vi "Receive Value Change Event.vi"(8 "error in (no error)":errorcluster, 10 "ValueChangeMsg":refnum<class "ValueChangeMsg.lvclass">, 11 "For Loop Dialog In":refnum<class "Test Step Dialog.lvclass">) -> (0 "error out":errorcluster, 3 "For Loop Dialog Out":refnum<class "Test Step Dialog.lvclass">)   [LabVIEW 2017, in "Test Step Dialog.lvclass"]
doc: "<License>\nCopyright © 2017 Composed Systems, LLC | All rights reserved\nwww.composed.io\n\nAuthor: Ethan Stern <ethan.stern@composed.io>\n\nThis software is provided \"AS IS\" WITHOUT WARRANTIES, either express or implied, AND IS FOR EDUCATIONAL PURPOSES ONLY.\n</License>"
uses:
  Test Step Dialog.lvclass
  C:/Program Files/National Instruments/LabVIEW 2017/vi.lib/ActorFramework/Actor/Actor.lvclass
  C:/Program Files/National Instruments/LabVIEW 2017/vi.lib/gpm_packages/@cs/popup-viewmanager/Source/Popup ViewManager/Popup ViewManager.lvclass
  D:/Test-executive-builder/Source/Test Executive Builder Dialogs/ITest Executive Builder Dialog/ITest Executive Builder Dialog.lvclass
  <vilib>/gpm_packages/@cs/mva-viewable/Source/ActorEvents/IEventAggregator Messages/ValueChangeMsg/ValueChangeMsg.lvclass
  <vilib>/gpm_packages/@cs/mva-viewable/Source/ActorEvents/IEventAggregator Messages/ValueChangeMsg/ValueChangeMsg.lvclass/ValueChangeMsg.ctl
  Data Type Handler/Test Executive Builder Data Type Handler.lvclass
  <vilib>/ActorFramework/Actor/Actor.lvclass/Actor.ctl
  <vilib>/ActorFramework/Message Enqueuer/Message Enqueuer.lvclass/Message Enqueuer.ctl
  Test Step Dialog.lvclass/Test Step Dialog.ctl
  <vilib>/gpm_packages/@cs/mva-viewable/Source/IViewable/IViewable Messages/Insert Front Panel Msg/Insert Front Panel Msg.lvclass/Insert Front Panel Msg.ctl
  IAttribute Data Type View Messages/Set Value Msg/Set Value Msg.lvclass/Set Value Msg.ctl
  ITest Executive Builder Dialog/ITest Executive Builder Dialog.lvclass/ITest Executive Builder Dialog.ctl
  698eee39-0e44-4932-ada2-d875f71f8c5a.vi
  7755fdff-7f77-4a95-a937-83a1493eaaf5.vi
  482c0f58-527f-4f41-8bf0-1e92f0d36b0a.vi
  <vilib>/ActorFramework/Message Enqueuer/Init from Existing Queue.vi
  <vilib>/ActorFramework/Message Enqueuer/Enqueue.vi
  ITest Executive Builder Dialog/Read Data Type Handler Type.vi
  <vilib>/Utility/error.llb/Clear Errors.vi
  <vilib>/ActorFramework/Stop Msg/Stop Msg.lvclass
  C:/Program Files/National Instruments/LabVIEW 2017/vi.lib/ActorFramework/Message/Message.lvclass
  <vilib>/gpm_packages/@cs/mva-viewable/Source/IViewable/IViewable Messages/Insert Front Panel Msg/Insert Front Panel Msg.lvclass
  IAttribute Data Type View Messages/Set Value Msg/Set Value Msg.lvclass
  <vilib>/ActorFramework/Message Priority Queue/Priority Enqueue.vi
  <vilib>/ActorFramework/Message Enqueuer/Message Enqueuer.lvclass
  <vilib>/gpm_packages/@cs/test-executive/Source/Test Executive/ITestExecutive/ITest Executive.lvclass
  ITest Executive Builder Dialog/ITest Executive Builder Dialog.lvclass
  <vilib>/ActorFramework/Actor/Actor.lvclass
  <vilib>/gpm_packages/@cs/popup-viewmanager/Source/Popup ViewManager/Popup ViewManager.lvclass
  <vilib>/gpm_packages/@cs/test-executive/Source/Test Executive/TestExecutive Ref/TestExecutive Ref.lvclass
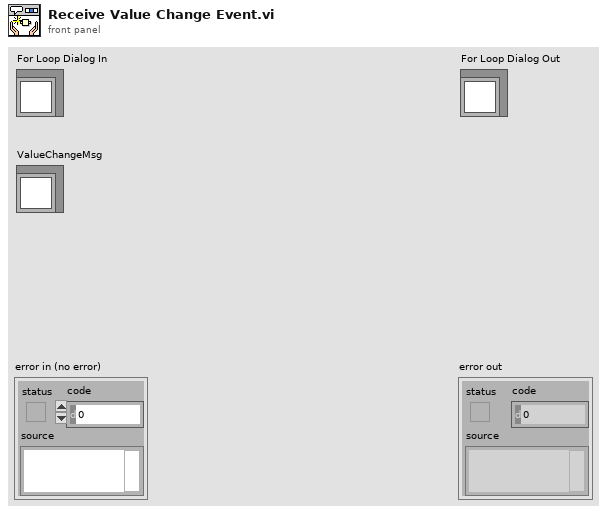
[diagram p1: front panel]
types:
  T1 = typedef "IViewable.lvlib/ProtectedSubpanel.lvclass/Protected Subpanel Reference.ctl" = refnum<data-value>
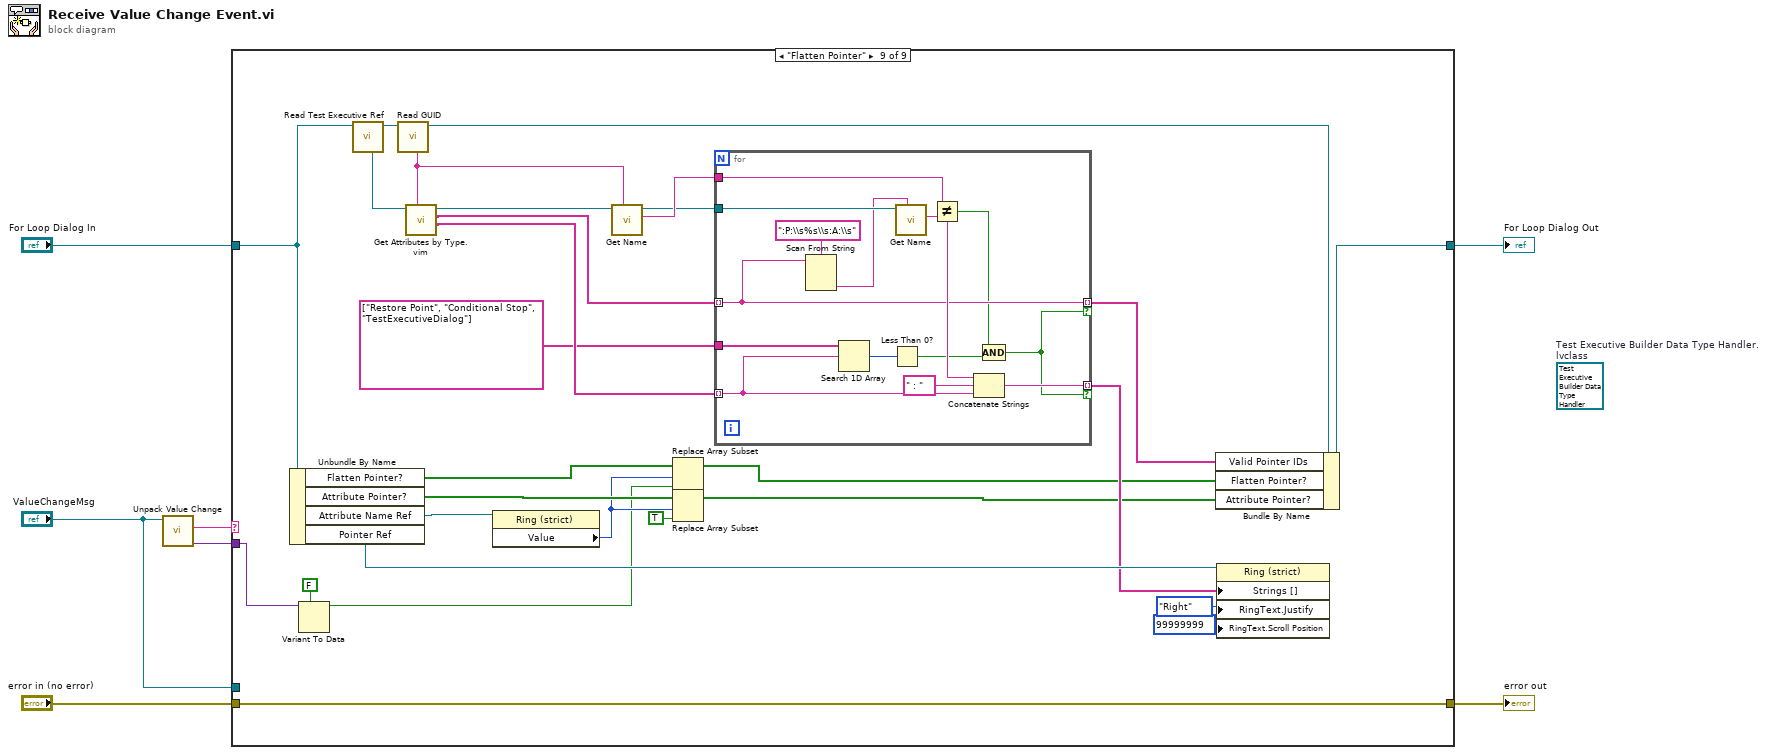
[diagram p0: block diagram]
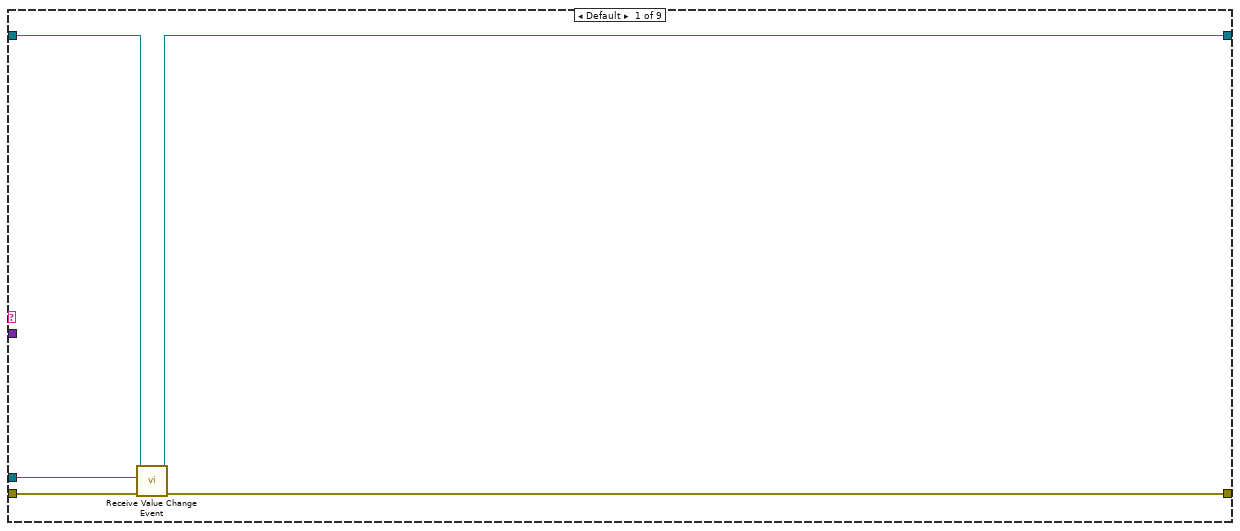
[diagram p2: hidden frame]
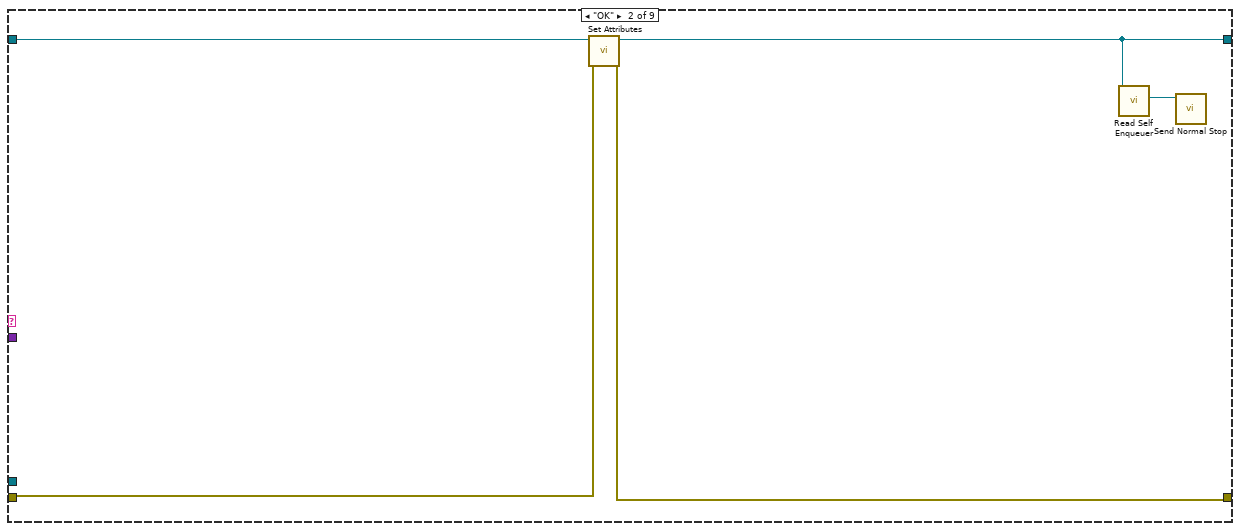
[diagram p3: hidden frame]
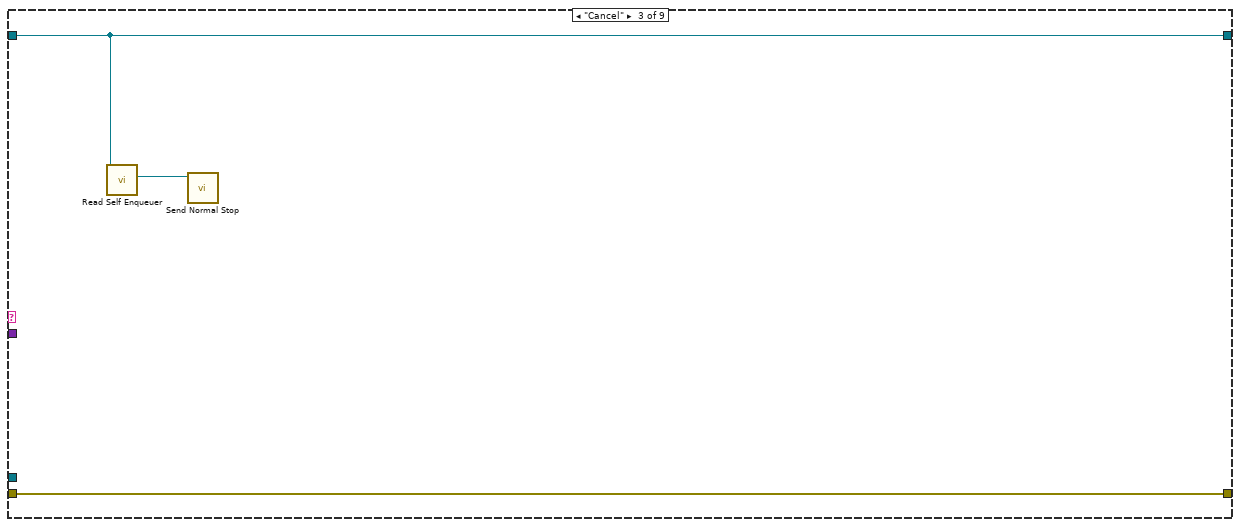
[diagram p4: hidden frame]
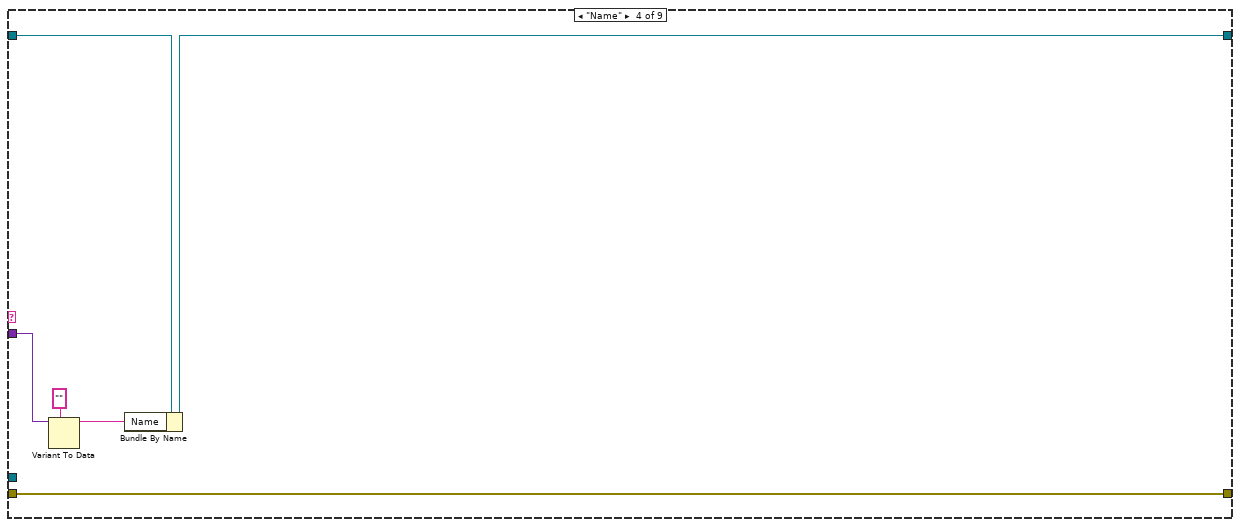
[diagram p5: hidden frame]
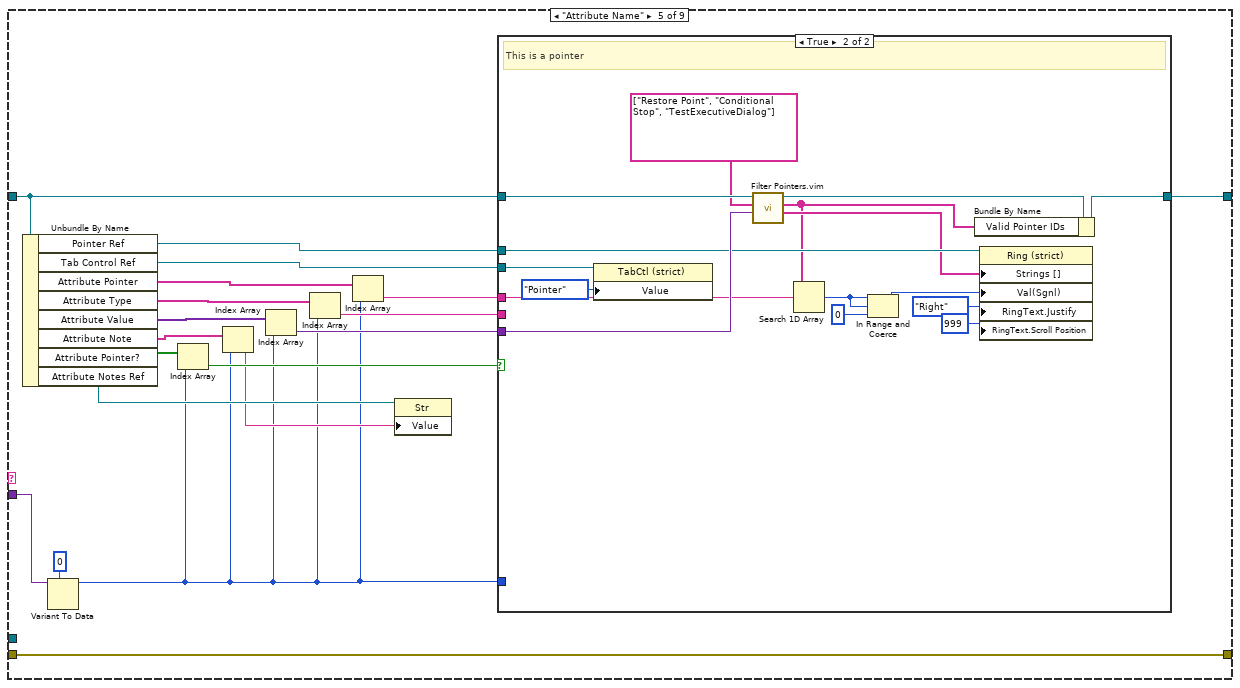
[diagram p6: hidden frame]
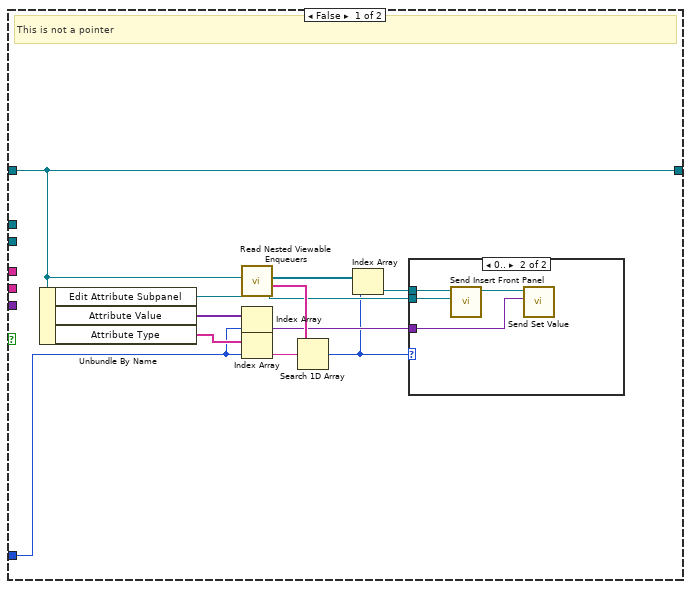
[diagram p7: hidden frame]
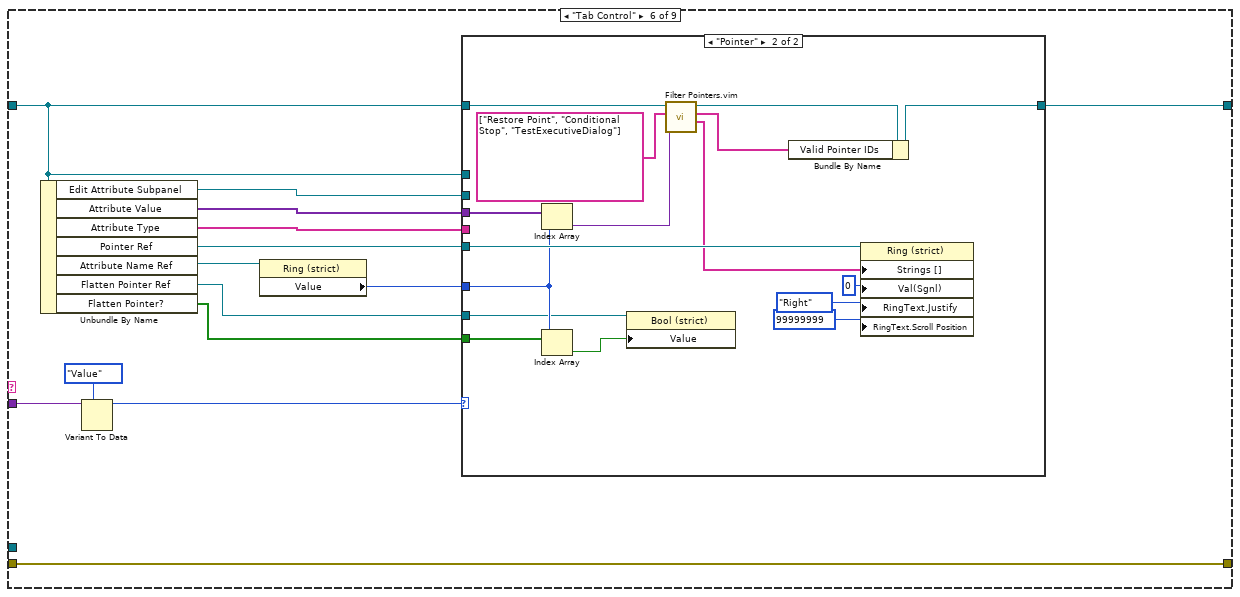
[diagram p9: hidden frame]
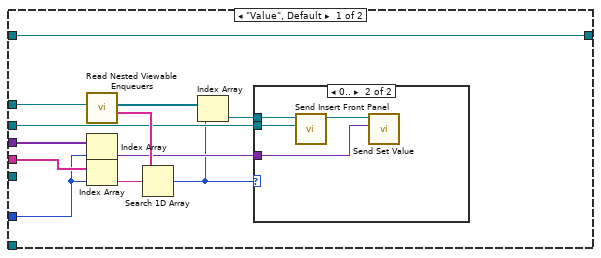
[diagram p10: hidden frame]
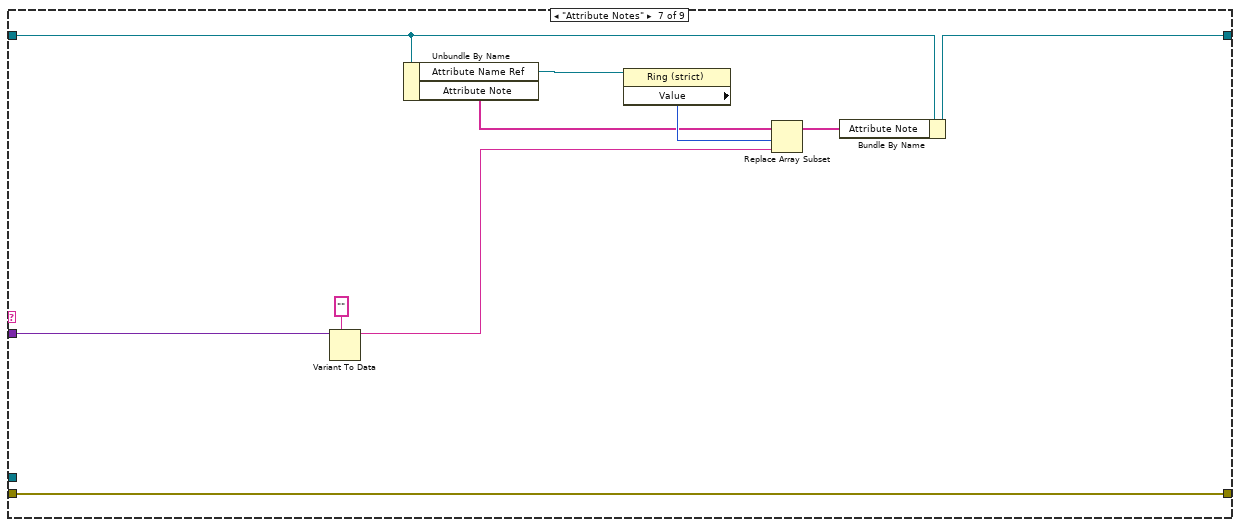
[diagram p12: hidden frame]
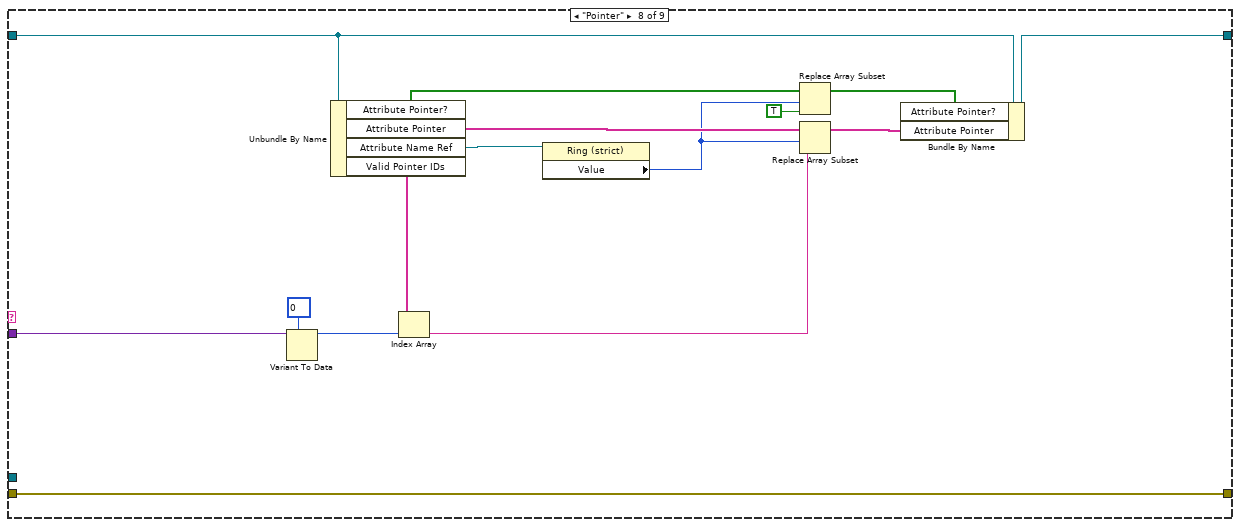
[diagram p13: hidden frame]
diagram:
  (unwired) refnum<class "Test Executive Builder Data Type Handler.lvclass"> refnum  # Test Executive Builder Data Type Handler.lvclass
  n1 = call <vilib>:"Unpack Value Change.vi"("ValueChangeMsg"="ValueChangeMsg") -> ("New Value"=w1:variant, "Control Label"=w2:string)  [unwired: 6 in, 3 out]
  n2 = case shown="\"Flatten Pointer\"" w2 {
    tunnel: [w12 w13 w20 w26 w45 w90 w132 w147 w175] -> w7
    tunnel: [w11 w15 w19 w21 w44 w86 w124 w134 w158] -> w6
    tunnel: "error in (no error)" -> [w10 w14 w20 w26 w45 w90 w132 w147 w175]
    tunnel: "For Loop Dialog In" -> [w9 w16 w19 w22 w43 w79 w125 w135 w173]
    tunnel: "ValueChangeMsg" -> [w8 _ _ _ _ _ _ _ _]
    tunnel: w1 -> [_ _ _ w25 w42 w89 w123 w133 w151]
    frame Default {
      n3 = call-parent "Receive Value Change Event.vi"("error in (no error)"=w10, "ValueChangeMsg"=w8, "IViewable In"=w9) -> ("error out"=w12:errorcluster, "IViewable Out"=w11:refnum<class "Test Step Dialog.lvclass">)  [unwired: 7 in]
    }
    frame "OK" {
      n4 = call-dynamic "Set Attributes.vi"("error in (no error)"=w14, "Test Step Dialog in"=w16) -> ("error out"=w13:errorcluster, "Test Step Dialog out"=w15:refnum<class "Test Step Dialog.lvclass">)  [unwired: 8 in]
      n5 = call <vilib>:"Read Self Enqueuer.vi"("Actor"=w15) -> ("Self Enqueuer"=w17:refnum<class "Message Enqueuer.lvclass">)  [unwired: 10 in]
      n6 = call <vilib>:"Send Normal Stop.vi"("Message Enqueuer"=w17) -> ()  [unwired: 10 in, 1 out]
    }
    frame "Cancel" {
      n7 = call <vilib>:"Read Self Enqueuer.vi"("Actor"=w19) -> ("Self Enqueuer"=w18:refnum<class "Message Enqueuer.lvclass">)  [unwired: 10 in]
      n8 = call <vilib>:"Send Normal Stop.vi"("Message Enqueuer"=w18) -> ()  [unwired: 10 in, 1 out]
    }
    frame "Name" {
      n9 = Variant To Data(type="" ("Iterations"), Variant=w25) -> (data=w23:string)  [unwired: 1 in, 1 out]
      n10 = Bundle By Name(cluster=w22, "Name"=w23) -> (w21:refnum<class "Test Step Dialog.lvclass">)
    }
    frame "Attribute Name" {
      n11 = Unbundle By Name(w43) -> ("Pointer Ref"=w30:refnum<vi>, "Tab Control Ref"=w31:refnum<vi>, "Attribute Pointer"=w36:string[], "Attribute Type"=w37:string[], "Attribute Value"=w38:variant[], "Attribute Note"=w39:string[], "Attribute Pointer?"=w40:bool[], "Attribute Notes Ref"=w29:refnum<vi>)
      n12 = Variant To Data(type=u16 0, Variant=w42) -> (data=w27:u16)  [unwired: 1 in, 1 out]
      n13 = Index Array(array=w40, index=w27) -> (element=w35:bool)
      n14 = Index Array(array=w39, index=w27) -> (element=w28:string)
      n15 = Index Array(array=w38, index=w27) -> (element=w34:variant)
      n16 = Index Array(array=w37, index=w27) -> (element=w33:string)
      n17 = Index Array(array=w36, index=w27) -> (element=w32:string)
      n18 = property class="Str"(reference=w29, "Value"=w28) -> ()  [unwired: 1 in, 2 out]
      n19 = case shown="True" w35 {
        tunnel: [w46 w67] -> w44
        tunnel: w43 -> [w46 w76]
        tunnel: w34 -> [_ w74]
        tunnel: w33 -> [_ _]
        tunnel: w32 -> [_ w65]
        tunnel: w31 -> [_ w73]
        tunnel: w30 -> [_ w72]
        tunnel: w27 -> [w47 _]
        frame False {
          # "This is not a pointer"
          n20 = Unbundle By Name(w46) -> ("Edit Attribute Subpanel"=w50:T1, "Attribute Value"=w55:variant[], "Attribute Type"=w56:string[])
          n21 = call <vilib>:"Read Nested Viewable Enqueuers.vi"("Popup ViewManager in"=w46) -> ("Viewable Names"=w52:string[], "Nested Enqueuers"=w54:refnum<class "Message Enqueuer.lvclass">[])  [unwired: 9 in]
          n22 = Index Array(array=w55, index=w47) -> (element=w49:variant)
          n23 = Index Array(array=w56, index=w47) -> (element=w51:string)
          n24 = Search 1D Array(1D array=w52, element=w51) -> (index of element=w48:i32)  [unwired: 1 in]
          n25 = Index Array(array=w54, index=w48) -> (element=w53:refnum<class "Message Enqueuer.lvclass">)
          n26 = case shown="0.." w48 {
            tunnel: w53 -> [_ w60]
            tunnel: w50 -> [_ w59]
            tunnel: w49 -> [_ w57]
            frame Default {
            }
            frame 0.. {
              n27 = call <vilib>:"Send Insert Front Panel.vi"("Protected Subpanel"=w59, "Message Enqueuer"=w60) -> ("Message Enqueuer out"=w58:refnum<class "Message Enqueuer.lvclass">)  [unwired: 8 in, 1 out]
              n28 = call "Send Set Value.vi"("Value"=w57, "Message Enqueuer"=w58) -> ()  [unwired: 8 in, 2 out]
            }
          }
        }
        frame True {
          # "This is a pointer"
          n29 = property class="TabCtl (strict)"(reference=w73, "Value"=enum32{"Value", "Pointer"}."Pointer") -> ()  [unwired: 1 in, 2 out]
          n30 = call "Filter Pointers.vim"("Type"=w74, "Exclusion List"=string[] ["Restore Point", "Conditional Stop", "TestExecutiveDialog"], "ITest Executive Builder Dialog in"=w76) -> ("Valid Pointer Names"=w69:string[], "Valid Pointer IDs"=w66:string[], "ITest Executive Builder Dialog out"=w68:refnum<class "Test Step Dialog.lvclass">)  [unwired: 5 in, 1 out]
          n31 = Search 1D Array(1D array=w66, element=w65) -> (index of element=w64:i32)  [unwired: 1 in]
          n32 = In Range and Coerce(upper limit=w64, x=w64, lower limit=0) -> (coerced(x)=w62:i32)  [unwired: 1 out]
          n33 = Bundle By Name(cluster=w68, "Valid Pointer IDs"=w66) -> (w67:refnum<class "Test Step Dialog.lvclass">)
          n34 = property class="Ring (strict)"(reference=w72, "Strings []"=w69, "Val(Sgnl)"=w62, "RingText.Justify"=enum16{"Left", "Center", "Right"}."Right" ("Ring Text.Justification"), "RingText.Scroll Position"=u32 999 ("Ring Text.Scroll Position")) -> ()  [unwired: 1 in, 2 out]
        }
      }
    }
    frame "Tab Control" {
      n35 = Unbundle By Name(w79) -> ("Edit Attribute Subpanel"=w85:T1, "Attribute Value"=w80:variant[], "Attribute Type"=w81:string[], "Pointer Ref"=w82:refnum<vi>, "Attribute Name Ref"=w87:refnum<vi>, "Flatten Pointer Ref"=w78:refnum<vi>, "Flatten Pointer?"=w77:bool[])
      n36 = Variant To Data(type=enum32{"Value", "Pointer"}."Value" ("Tab Control"), Variant=w89) -> (data=w84:enum32{"Value", "Pointer"})  [unwired: 1 in, 1 out]
      n37 = property class="Ring (strict)"(reference=w87) -> ("Value"=w83:u16)  [unwired: 1 in, 2 out]
      n38 = case shown="\"Pointer\"" w84 {
        tunnel: w81 -> [w102 _]
        tunnel: w80 -> [w101 w121]
        tunnel: w85 -> [w96 _]
        tunnel: w79 -> [w94 _]
        tunnel: w83 -> [w93 w109]
        tunnel: [w91 w115] -> w86
        tunnel: w79 -> [w91 w122]
        tunnel: w82 -> [_ w118]
        tunnel: w78 -> [_ w108]
        tunnel: w77 -> [_ w110]
        frame "Value", Default {
          n39 = call <vilib>:"Read Nested Viewable Enqueuers.vi"("Popup ViewManager in"=w94) -> ("Viewable Names"=w98:string[], "Nested Enqueuers"=w100:refnum<class "Message Enqueuer.lvclass">[])  [unwired: 9 in]
          n40 = Index Array(array=w101, index=w93) -> (element=w95:variant)
          n41 = Index Array(array=w102, index=w93) -> (element=w97:string)
          n42 = Search 1D Array(1D array=w98, element=w97) -> (index of element=w92:i32)  [unwired: 1 in]
          n43 = Index Array(array=w100, index=w92) -> (element=w99:refnum<class "Message Enqueuer.lvclass">)
          n44 = case shown="0.." w92 {
            tunnel: w99 -> [_ w106]
            tunnel: w96 -> [_ w105]
            tunnel: w95 -> [_ w103]
            frame Default {
            }
            frame 0.. {
              n45 = call <vilib>:"Send Insert Front Panel.vi"("Protected Subpanel"=w105, "Message Enqueuer"=w106) -> ("Message Enqueuer out"=w104:refnum<class "Message Enqueuer.lvclass">)  [unwired: 8 in, 1 out]
              n46 = call "Send Set Value.vi"("Value"=w103, "Message Enqueuer"=w104) -> ()  [unwired: 8 in, 2 out]
            }
          }
        }
        frame "Pointer" {
          n47 = Index Array(array=w121, index=w109) -> (element=w120:variant)
          n48 = Index Array(array=w110, index=w109) -> (element=w107:bool)
          n49 = property class="Bool (strict)"(reference=w108, "Value"=w107) -> ()  [unwired: 1 in, 2 out]
          n50 = call "Filter Pointers.vim"("Type"=w120, "Exclusion List"=string[] ["Restore Point", "Conditional Stop", "TestExecutiveDialog"], "ITest Executive Builder Dialog in"=w122) -> ("Valid Pointer Names"=w117:string[], "Valid Pointer IDs"=w114:string[], "ITest Executive Builder Dialog out"=w116:refnum<class "Test Step Dialog.lvclass">)  [unwired: 5 in, 1 out]
          n51 = Bundle By Name(cluster=w116, "Valid Pointer IDs"=w114) -> (w115:refnum<class "Test Step Dialog.lvclass">)
          n52 = property class="Ring (strict)"(reference=w118, "Strings []"=w117, "Val(Sgnl)"=u16 0 ("Value (Signaling)"), "RingText.Justify"=enum16{"Left", "Center", "Right"}."Right" ("Ring Text.Justification"), "RingText.Scroll Position"=u32 99999999 ("Ring Text.Scroll Position")) -> ()  [unwired: 1 in, 2 out]
        }
      }
    }
    frame "Attribute Notes" {
      n53 = Variant To Data(type="", Variant=w123) -> (data=w127:string)  [unwired: 1 in, 1 out]
      n54 = Unbundle By Name(w125) -> ("Attribute Name Ref"=w131:refnum<vi>, "Attribute Note"=w129:string[])
      n55 = property class="Ring (strict)"(reference=w131) -> ("Value"=w130:u16)  [unwired: 1 in, 2 out]
      n56 = Replace Array Subset(array=w129, new element=w127, index=w130) -> (w126:string[])
      n57 = Bundle By Name(cluster=w125, "Attribute Note"=w126) -> (w124:refnum<class "Test Step Dialog.lvclass">)
    }
    frame "Pointer" {
      w146 = u16 0 items=[""] ("Pointer")
      n58 = Variant To Data(type=w146, Variant=w133) -> (data=w138:u16)  [unwired: 1 in, 1 out]
      n59 = Unbundle By Name(w135) -> ("Attribute Pointer?"=w143:bool[], "Attribute Pointer"=w144:string[], "Attribute Name Ref"=w145:refnum<vi>, "Valid Pointer IDs"=w137:string[])
      n60 = Index Array(array=w137, index=w138) -> (element=w136:string)
      n61 = property class="Ring (strict)"(reference=w145) -> ("Value"=w142:u16)  [unwired: 1 in, 2 out]
      n62 = Replace Array Subset(array=w143, new element=TRUE ("new element/subarray"), index=w142) -> (w139:bool[])
      n63 = Replace Array Subset(array=w144, new element=w136, index=w142) -> (w140:string[])
      n64 = Bundle By Name(cluster=w135, "Attribute Pointer?"=w139, "Attribute Pointer"=w140) -> (w134:refnum<class "Test Step Dialog.lvclass">)
    }
    frame "Flatten Pointer" {
      n65 = Unbundle By Name(w173) -> ("Flatten Pointer?"=w153:bool[], "Attribute Pointer?"=w156:bool[], "Attribute Name Ref"=w164:refnum<vi>, "Pointer Ref"=w163:refnum<vi>)
      n66 = Variant To Data(type=FALSE, Variant=w151) -> (data=w149:bool)  [unwired: 1 in, 1 out]
      n67 = call "Read Test Executive Ref.vi"("ITest Executive Builder Dialog in"=w173) -> ("ITest Executive Builder Dialog out"=w174:refnum<class "Test Step Dialog.lvclass">, "Test Executive Ref"=w172:refnum<data-value>)  [unwired: 9 in]
      n68 = call "Read GUID.vi"("ITest Executive Builder Dialog in"=w174) -> ("ITest Executive Builder Dialog out"=w159:refnum<class "Test Step Dialog.lvclass">, "GUID"=w168:string)  [unwired: 9 in]
      n69 = call "Get Attributes by Type.vim"("ID"=w168, "Test Executive Ref"=w172) -> ("Names"=w166:string[], "IDs"=w167:string[], "Test Executive Ref out"=w169:refnum<data-value>)  [unwired: 5 in, 2 out]
      n70 = property class="Ring (strict)"(reference=w164) -> ("Value"=w152:u16)  [unwired: 1 in, 2 out]
      n71 = call <vilib>:"Get Name.vi"("Unique ID"=w168, "Test Executive Ref"=w169) -> ("Name"=w171:string, "Test Executive Ref out"=w170:refnum<data-value>)  [unwired: 5 in, 3 out]
      n72 = Replace Array Subset(array=w153, new element=w149, index=w152) -> (w148:bool[])
      n73 = Replace Array Subset(array=w156, new element=TRUE ("new element/subarray"), index=w152) -> (w154:bool[])
      n74 = for {
        tunnel: w166 -> [w181] mode=indexing
        tunnel: w167 -> [w182] mode=indexing
        tunnel: w171 -> [w186]
        tunnel: w170 -> [w188]
        tunnel: [w183] -> w162 mode=indexing if=w176
        tunnel: [w182] -> w157 mode=indexing if=w176
        tunnel: string[] ["Restore Point", "Conditional Stop", "TestExecutiveDialog"] ("Exclusion List") -> [w180]
        n75 = Scan From String(format string=":P:\\s%s\\s:A:\\s", input string=w182) -> (output 1=w187:string)  [unwired: 3 in, 3 out]
        n76 = Search 1D Array(1D array=w180, element=w181) -> (index of element=w179:i32)  [unwired: 1 in]
        n77 = Less Than 0?(x=w179) -> (x < 0?=w178:bool)
        n78 = call <vilib>:"Get Name.vi"("Unique ID"=w187, "Test Executive Ref"=w188) -> ("Name"=w184:string)  [unwired: 5 in, 4 out]
        n79 = Not Equal?(x=w186, y=w184) -> (x != y?=w177:bool)
        n80 = Concatenate Strings(w184, " : " ("string"), w181) -> (w183:string)
        n81 = Compound Arithmetic op=AND(w177, w178) -> (w176:bool)
      }
      n82 = Bundle By Name(cluster=w159, "Valid Pointer IDs"=w157, "Flatten Pointer?"=w148, "Attribute Pointer?"=w154) -> (w158:refnum<class "Test Step Dialog.lvclass">)
      n83 = property class="Ring (strict)"(reference=w163, "Strings []"=w162, "RingText.Justify"=enum16{"Left", "Center", "Right"}."Right" ("Ring Text.Justification"), "RingText.Scroll Position"=u32 99999999 ("Ring Text.Scroll Position")) -> ()  [unwired: 1 in, 2 out]
    }
  }
  "error out" <- w7
  "For Loop Dialog Out" <- w6
